vi "Write T string.vi"(8 "error in (no error)":errorcluster, 10 "T string":string="T", 11 "Bool D Element in":refnum<class "Bool D Element.lvclass">) -> (0 "error out":errorcluster, 3 "Bool D Element out":refnum<class "Bool D Element.lvclass">)   [LabVIEW 2020, in "D Datagrid Library.lvlib" / "Bool D Element.lvclass"]
uses:
  Bool D Element.lvclass
  Bool D Element.lvclass/Bool D Element.ctl
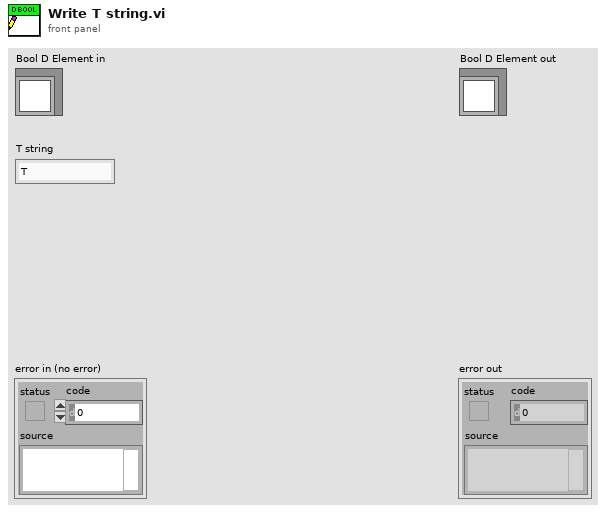
[diagram p1: front panel]
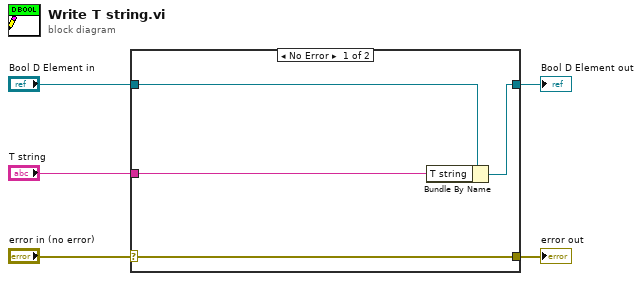
[diagram p0: block diagram]
diagram:
  n1 = case shown="No Error" "error in (no error)" {
    selector: "error in (no error)" -> [w9 w10]
    tunnel: [w9 w10] -> w4
    tunnel: [w7 w11] -> w2
    tunnel: "Bool D Element in" -> [w8 w11]
    tunnel: "T string" -> [w6 _]
    frame No Error {
      n2 = Bundle By Name(cluster=w8, "T string"=w6) -> (w7:refnum<class "Bool D Element.lvclass">)
    }
    frame Error {
    }
  }
  "error out" <- w4
  "Bool D Element out" <- w2
